vi "Edge-Plane intersection test.vi"(2 "Plane normal (unit)":sgl[](array[numeric]), 3 "Point on plane":sgl[](array[numeric]), 4 "Edge vector (not unit)":sgl[](array[numeric]), 5 "Edge start point":sgl[](array[numeric])) -> (0 "Intersection point":sgl[](array[numeric]), 1 "Intersection":bool)   [LabVIEW 2014]
panel:
  # "PN 13/01/2015"
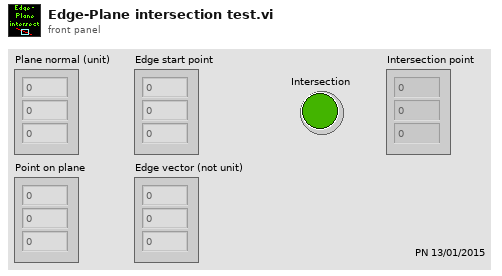
[diagram p1: front panel]
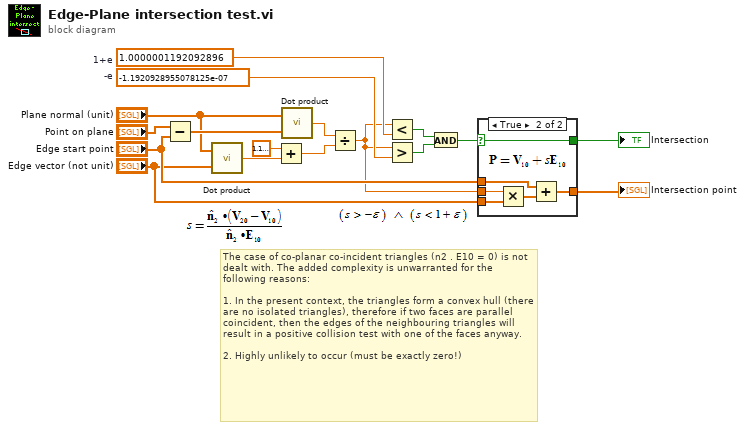
[diagram p0: block diagram]
diagram:
  w13 = sgl -1.1920929e-07  # -e
  w14 = sgl 1.0000001  # 1+e
  # "The case of co-planar co-incident triangles (n2 . E10 = 0) is not dealt with. The added complexity is unwarranted for the following reasons:\n\n1. In the present context, the triangles form a convex hull (there are no isolated triangles), therefore if two faces are parallel coincident, then the edges of the neighbouring triangles will result in a positive collision test with one of the faces anyway.\n\n2. Highly unlikely to occur (must be exactly zero!)"
  n1 = Subtract(x="Point on plane", y="Edge start point") -> (x-y=w16:sgl[])
  n2 = call "Dot product.vi"("B"="Edge vector (not unit)", "A"="Plane normal (unit)") -> ("A . B"=w2:sgl)
  n3 = Add(x=sgl 1.1920929e-07, y=w2) -> (x+y=w3:sgl)
  n4 = call "Dot product.vi"("B"=w16, "A"="Plane normal (unit)") -> ("A . B"=w6:sgl)
  n5 = Divide(x=w6, y=w3) -> (x/y=w4:sgl)
  n6 = Less?(x=w4, y=w14) -> (x < y?=w7:bool)
  n7 = Greater?(x=w4, y=w13) -> (0:w8:bool)
  n8 = And(x=w7, y=w8) -> (x .and. y?=w5:bool)
  n9 = case shown="True" w5 {
    selector: w5 -> [w18 w24]
    tunnel: [w18 w24] -> w12
    tunnel: w4 -> [_ w23]
    tunnel: "Edge start point" -> [_ w21]
    tunnel: "Edge vector (not unit)" -> [_ w22]
    tunnel: [_ w19] -> w9
    frame False {
    }
    frame True {
      n10 = Multiply(x=w23, y=w22) -> (x*y=w20:sgl[])
      n11 = Add(x=w21, y=w20) -> (x+y=w19:sgl[])
    }
  }
  "Intersection point" <- w9
  "Intersection" <- w12
